vi "Autonomous Global Data.vi"() -> ()   [LabVIEW 2012]
panel:
  in  "Auto Type":u16 max=1 step=1
  in  "Auto Modet":u16 max=10 step=1
  in  "R3":dbl min=-1.0 max=1.0 step=0.01
  in  "R2":dbl=-0.6499999999999997 min=-1.0 max=1.0 step=0.01
  in  "R1":dbl=-0.6499999999999997 min=-1.0 max=1.0 step=0.01
  in  "D3":dbl min=0.0 max=12.0 step=0.01
  in  "D2":dbl=4.049999999999999 min=0.0 max=12.0 step=0.01
  in  "D1":dbl=4.51 min=0.0 max=12.0 step=0.01
  in  "COV Waito":dbl=4000.0 max=10000.0 step=100.0
  in  "COV Speede":dbl=-0.5 max=1.0 step=0.01
  # "Key Shoot\n1 = Yes\n0 = No"
  # "0= three point\n1= two point"
  # "Disance to Travel"
  # "Rate to tavel at"
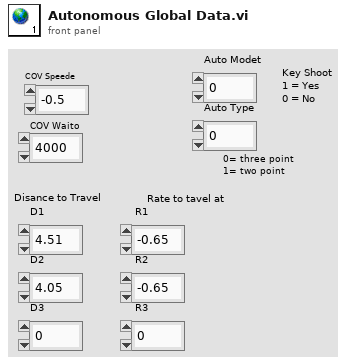
[diagram p1: front panel]
diagram:
